vi "Action Select Instrument.vi"(0 "VISA resource name":refnum<visa-resource-name>, 5 "Logical Instrument Name":string, 7 "Logical Instrument Number":u32, 11 "error in (no error)":errorcluster) -> (4 "VISA resource name out":refnum<visa-resource-name>, 15 "error out":errorcluster)   [LabVIEW 2020, in "NH Research Regenerative Test Series.lvlib"]
doc: "Selects an instrument as the default. If <B>Logical Instrument Name</B> is provided, then <B>Logical Instrument Number</B> will be ignored and the instrument will be selected by the name string input. If the <B>Logical Instrument Name</B> string is blank, then the instrument will be selected by the instrument number provided in <B>Logical Instrument Number</B>.\n\nBy selecting an instrument by name and then querying the selected instrument by name, the equivalence between the instrument number and identifier can be determined. For example, by selecting a logical instrument by name with this VI and then querying which logical instrument is selected with the Query Selected Instrument, the corresponding numeric value shall be returned.\n\nNOTE: The 4900 only has one logical instrument so the only valid instrument number is 1."
uses:
  NH Research Regenerative Test Series.lvlib
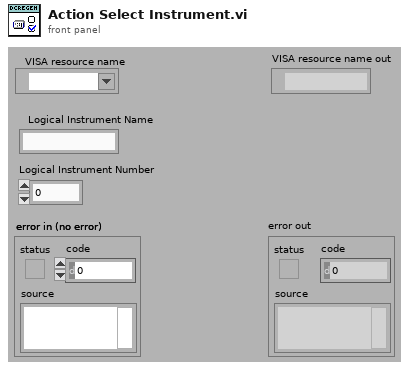
[diagram p1: front panel]
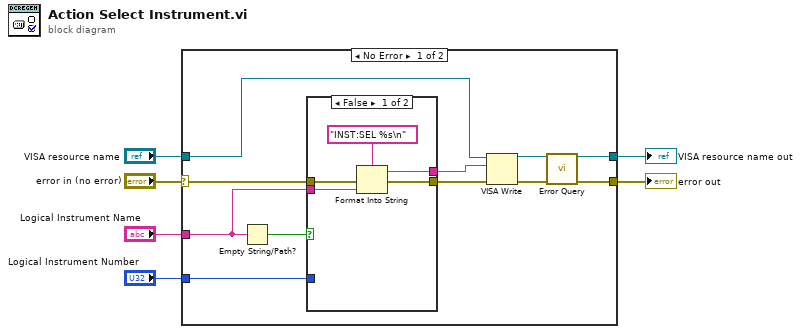
[diagram p0: block diagram]
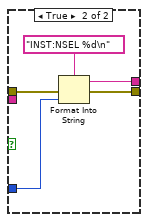
[diagram p2: hidden frame]
diagram:
  n1 = case shown="No Error" "error in (no error)" {
    selector: "error in (no error)" -> [w14 w29]
    tunnel: "VISA resource name" -> [w9 w28]
    tunnel: [w16 w28] -> w5
    tunnel: [w15 w29] -> w4
    tunnel: "Logical Instrument Name" -> [w8 _]
    tunnel: "Logical Instrument Number" -> [w7 _]
    frame No Error {
      n2 = Empty String/Path?(string/path=w8) -> (empty?=w10:bool)
      n3 = case shown="False" w10 {
        tunnel: [w21 w26] -> w17
        tunnel: w14 -> [w20 w25]
        tunnel: [w19 w24] -> w13
        tunnel: w8 -> [w18 _]
        tunnel: w7 -> [_ w23]
        frame False {
          n4 = Format Into String(format string="INST:SEL %s\n" ("Command"), error in=w20, w18) -> (resulting string=w21:string, error out=w19:errorcluster)  [unwired: 1 in]
        }
        frame True {
          n5 = Format Into String(format string="INST:NSEL %d\n" ("Command"), error in=w25, w23) -> (resulting string=w26:string, error out=w24:errorcluster)  [unwired: 1 in]
        }
      }
      n6 = VISA Write(VISA resource name=w9, write buffer=w17, error in (no error)=w13) -> (VISA resource name out=w12:refnum<visa-resource-name>, error out=w11:errorcluster)  [unwired: 1 out]
      n7 = call "Error Query.vi"("VISA resource name"=w12, "error in (no error)"=w11) -> ("VISA resource name out"=w16:refnum<visa-resource-name>, "error out"=w15:errorcluster)  [unwired: 10 in, 2 out]
    }
    frame Error {
    }
  }
  "error out" <- w4
  "VISA resource name out" <- w5
